vi "niDTS WLAN INSTR TX Configure PortManagement.vi"(8 "error in (no error)":errorcluster, 11 "niDTS WLAN INSTR TX in":refnum<class "niDTS WLAN INSTR TX.lvclass">) -> (0 "error out":errorcluster, 3 "niDTS WLAN INSTR TX out":refnum<class "niDTS WLAN INSTR TX.lvclass">)   [LabVIEW 2015, in "niDTS WLAN.lvlib" / "niDTS WLAN INSTR TX.lvclass"]
uses:
  niDTS WLAN INSTR TX.lvclass
  niDTS WLAN INSTR TX.lvclass/niDTS WLAN INSTR TX.ctl
  RiviInstDriver/niRfsaWlan/Objects/niRfsaWlan.lvclass
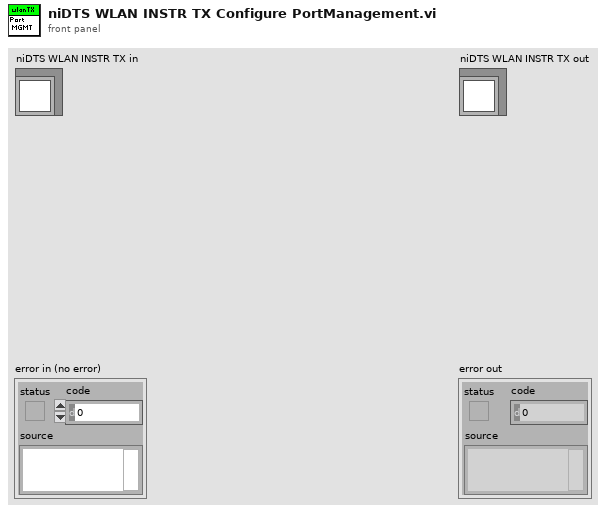
[diagram p1: front panel]
types:
  T1 = typedef "niRfsaWlan.lvclass/niRfsaWlan INC Handle.ctl" = refnum<data-value>
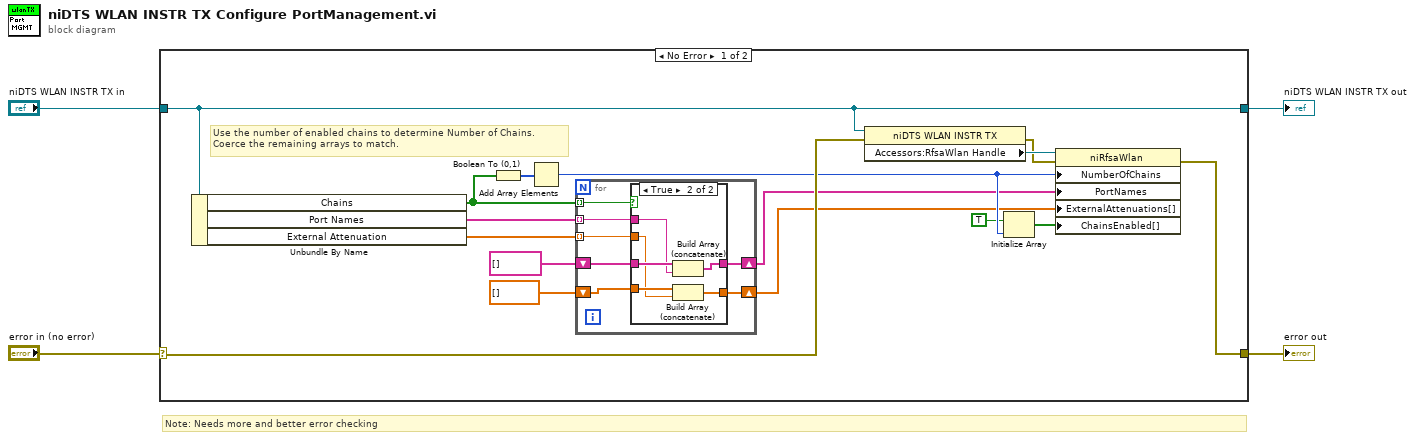
[diagram p0: block diagram]
diagram:
  # "Note: Needs more and better error checking"
  n1 = case shown="No Error" "error in (no error)" {
    selector: "error in (no error)" -> [w19 w37]
    tunnel: [w16 w37] -> w3
    tunnel: [w20 w36] -> w1
    tunnel: "niDTS WLAN INSTR TX in" -> [w20 w36]
    frame No Error {
      # "Use the number of enabled chains to determine Number of Chains.\nCoerce the remaining arrays to match."
      n2 = Unbundle By Name(w20) -> ("Chains"=w14:bool[], "Port Names"=w13:string[], "External Attenuation"=w12:dbl[])
      n3 = Boolean To (0,1)(Boolean=w14) -> (0, 1=w15:i16[])
      n4 = Add Array Elements(numeric array=w15) -> (sum=w9:i16)
      n5 = for {
        tunnel: w14 -> [w27] mode=indexing
        tunnel: w13 -> [w21] mode=indexing
        tunnel: w12 -> [w26] mode=indexing
        shift-right: [w23] -> w6
        shift-left: string[] [] ("Port Names") -> [w25]
        shift-right: [w22] -> w5
        shift-left: dbl[] [] ("WLAN Tx Input Parameters.External Attenuation") -> [w24]
        n6 = case shown="True" w27 {
          tunnel: w21 -> [_ w32]
          tunnel: w26 -> [_ w33]
          tunnel: w25 -> [w29 w35]
          tunnel: w24 -> [w28 w34]
          tunnel: [w29 w31] -> w23
          tunnel: [w28 w30] -> w22
          frame False {
          }
          frame True {
            n7 = Build Array (concatenate)(w35, w32) -> (w31:string[])
            n8 = Build Array (concatenate)(w34, w33) -> (w30:dbl[])
          }
        }
      }
      n9 = property class="niDTS WLAN INSTR TX"(reference=w20, error in=w19) -> (error out=w17:errorcluster, "Accessors:RfsaWlan Handle"=w18:T1)  [unwired: 1 out]
      n10 = Initialize Array(TRUE, w9) -> (w7:bool[])
      n11 = property class="niRfsaWlan"(reference=w18, error in=w17, "NumberOfChains"=w9, "PortNames"=w6, "ExternalAttenuations[]"=w5, "ChainsEnabled[]"=w7) -> (error out=w16:errorcluster)  [unwired: 1 out]
    }
    frame Error {
    }
  }
  "error out" <- w3
  "niDTS WLAN INSTR TX out" <- w1
